vi "Log.vi"(8 "error in (no error)":errorcluster, 10 "LogRecord":refnum<class "LogRecord.lvclass">, 11 "SQLiteLogHandle in":refnum<class "SQLiteLogHandle.lvclass">) -> (0 "error out":errorcluster, 3 "SQLiteLogHandle out":refnum<class "SQLiteLogHandle.lvclass">)   [LabVIEW 2024, in "SQLiteLogHandle.lvclass"]
uses:
  SQLiteLogHandle.lvclass
  Record/LogRecord.lvclass
  SQLiteLogHandle.lvclass/SQLiteLogHandle.ctl
  <vilib>/drjdpowell/SQLite Library/SQL Statement/SQL Statement.lvclass
  <vilib>/drjdpowell/SQLite Library/Transaction Helpers/Transaction.lvlib
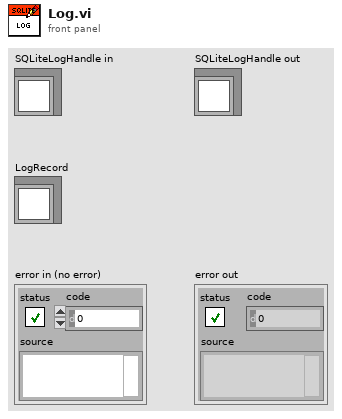
[diagram p1: front panel]
types:
  T1 = typedef "LoggerShared.lvlib/Level.ctl" = enum16{"DEBUG", "INFO", "WARNING", "ERROR", "CRITICAL"}
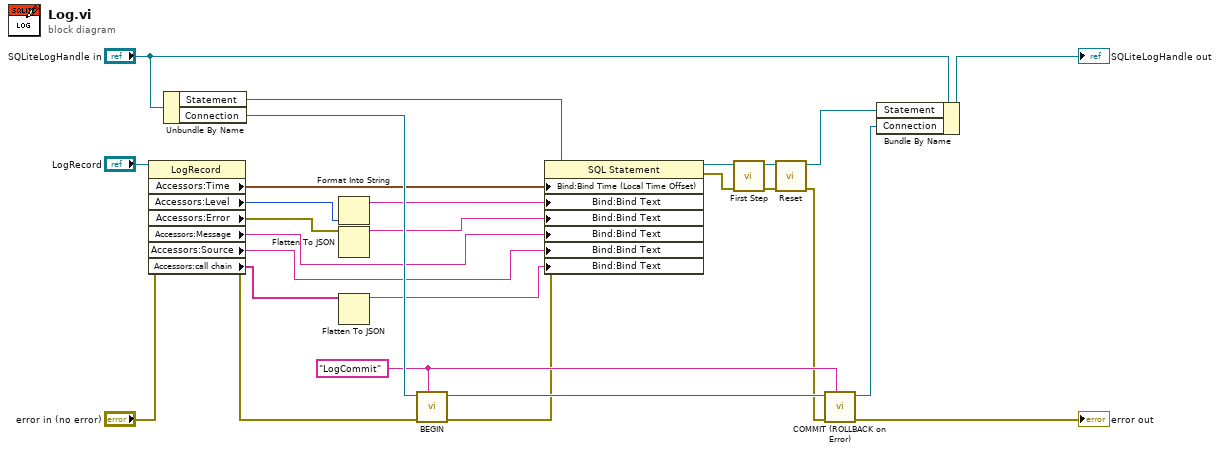
[diagram p0: block diagram]
diagram:
  w21 = "LogCommit" ("Savepoint name")
  n1 = property class="LogRecord"(reference="LogRecord", error in="error in (no error)") -> (error out=w25:errorcluster, "Accessors:Time"=w9:timestamp, "Accessors:Level"=w8:T1, "Accessors:Error"=w6:errorcluster, "Accessors:Message"=w4:string, "Accessors:Source"=w3:string, "Accessors:call chain"=w2:string[])  [unwired: 1 out]
  n2 = Unbundle By Name("SQLiteLogHandle in") -> ("Statement"=w11:refnum<class "SQL Statement.lvclass">, "Connection"=w24:refnum<class "Connection.lvclass">)
  n3 = Format Into String(w8) -> (resulting string=w7:string)  [unwired: 3 in, 1 out]
  n4 = Flatten To JSON(anything=w6) -> (JSON string=w5:string)  [unwired: 2 in, 1 out]
  n5 = Flatten To JSON(anything=w2) -> (JSON string=w1:string)  [unwired: 2 in, 1 out]
  n6 = call <vilib>:"BEGIN.vi"("Savepoint name"=w21, "error in (no error)"=w25, "SQLite Connection in"=w24) -> ("error out"=w17:errorcluster, "SQLite Connection"=w22:refnum<class "Connection.lvclass">)  [unwired: 7 in]
  n7 = property class="SQL Statement"(reference=w11, error in=w17, "Bind:Bind Time (Local Time Offset)"=w9, "Bind:Bind Text"=w7, "Bind:Bind Text"=w5, "Bind:Bind Text"=w4, "Bind:Bind Text"=w3, "Bind:Bind Text"=w1) -> (reference out=w10:refnum<class "SQL Statement.lvclass">, error out=w12:errorcluster)
  n8 = call <vilib>:"First Step.vi"("error in (no error)"=w12, "SQL Statement in"=w10) -> ("error out"=w16:errorcluster, "SQL Statement"=w15:refnum<class "SQL Statement.lvclass">)  [unwired: 7 in, 1 out]
  n9 = call <vilib>:"Reset.vi"("error in (no error)"=w16, "SQL Statement in"=w15) -> ("error out"=w14:errorcluster, "SQL Statement"=w13:refnum<class "SQL Statement.lvclass">)  [unwired: 8 in]
  n10 = call <vilib>:"COMMIT (ROLLBACK on Error).vi"("Savepoint name"=w21, "error in (no error)"=w14, "SQLite Connection in"=w22) -> ("error out"=→"error out":errorcluster, "SQLite Connection"=w18:refnum<class "Connection.lvclass">)  [unwired: 7 in]
  n11 = Bundle By Name(cluster="SQLiteLogHandle in", "Statement"=w13, "Connection"=w18) -> (→"SQLiteLogHandle out":refnum<class "SQLiteLogHandle.lvclass">)
